vi "Handle File List.vi"(10 "Source":enum32{"Files", "Camera"}(ring), 11 "Folder Location in":path) -> (1 "force":bool, 2 "filenames":string[](array[string]), 3 "Folder Location out":path)   [LabVIEW 2019]
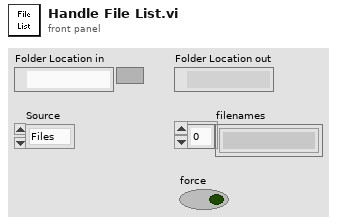
[diagram p1: front panel]
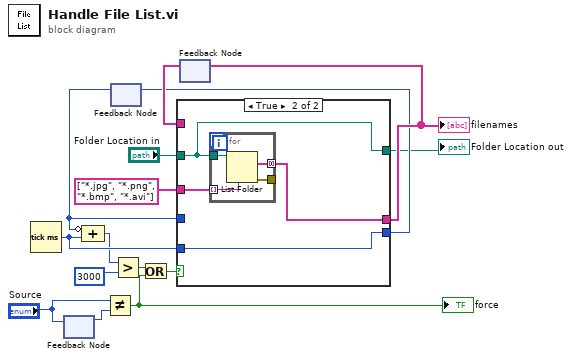
[diagram p0: block diagram]
diagram:
  n1 = Tick Count (ms)() -> (millisecond timer value=w9:u32)
  n2 = feedback #1() -> (w7:enum32{"Files", "Camera"})  [unwired: 1 in]
  n3 = feedback-in #1("Source") -> ()
  n4 = Not Equal?(x="Source", y=w7) -> (x != y?=w15:bool)
  "force" <- w15
  n5 = feedback #2() -> (w10:u32)  [unwired: 1 in]
  n6 = Compound Arithmetic op=ADD(invert w10, w9) -> (w6:u32)
  n7 = Greater?(x=w6, y=u32 3000 ("delay (ms)")) -> (0:w5:bool)
  n8 = Or(x=w5, y=w15) -> (x .or. y?=w11:bool)
  n9 = feedback #3() -> (w13:string[])  [unwired: 1 in]
  n10 = case shown="True" w11 {
    tunnel: w9 -> [_ w22]
    tunnel: [w18 w22] -> w8
    tunnel: w10 -> [w18 _]
    tunnel: string[] ["*.jpg", "*.png", "*.bmp", "*.avi"] -> [_ w21]
    tunnel: "Folder Location in" -> [w17 w20]
    tunnel: [w17 w20] -> w2
    tunnel: w13 -> [w16 _]
    tunnel: [w16 w19] -> w14
    frame False {
    }
    frame True {
      n11 = for {
        tunnel: [w26] -> w19 mode=concatenating
        tunnel: w20 -> [w25]
        tunnel: [w24] -> _
        tunnel: w21 -> [w23] mode=indexing
        n12 = List Folder(path=w25, pattern=w23) -> (filenames=w26:string[], error out=w24:errorcluster)  [unwired: 2 in, 2 out]
      }
    }
  }
  "filenames" <- w14
  "Folder Location out" <- w2
  n13 = feedback-in #2(w8) -> ()
  n14 = feedback-in #3(w14) -> ()
